vi "Multiplot-Disable.vi"() -> ()   [LabVIEW 2014]
uses:
  Stop.ctl
panel:
  in  "stop":T1
  in  "OK Button 3":bool
  in  "OK Button 2":bool
  in  "OK Button":bool
  out "Waveform Graph":dynamicdata(graph)
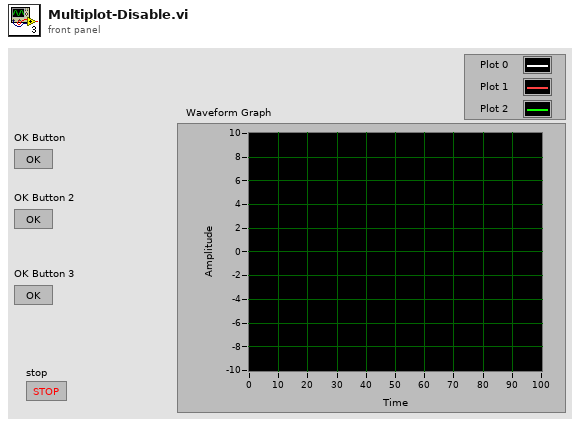
[diagram p1: front panel]
types:
  T1 = typedef "Stop.ctl" = bool
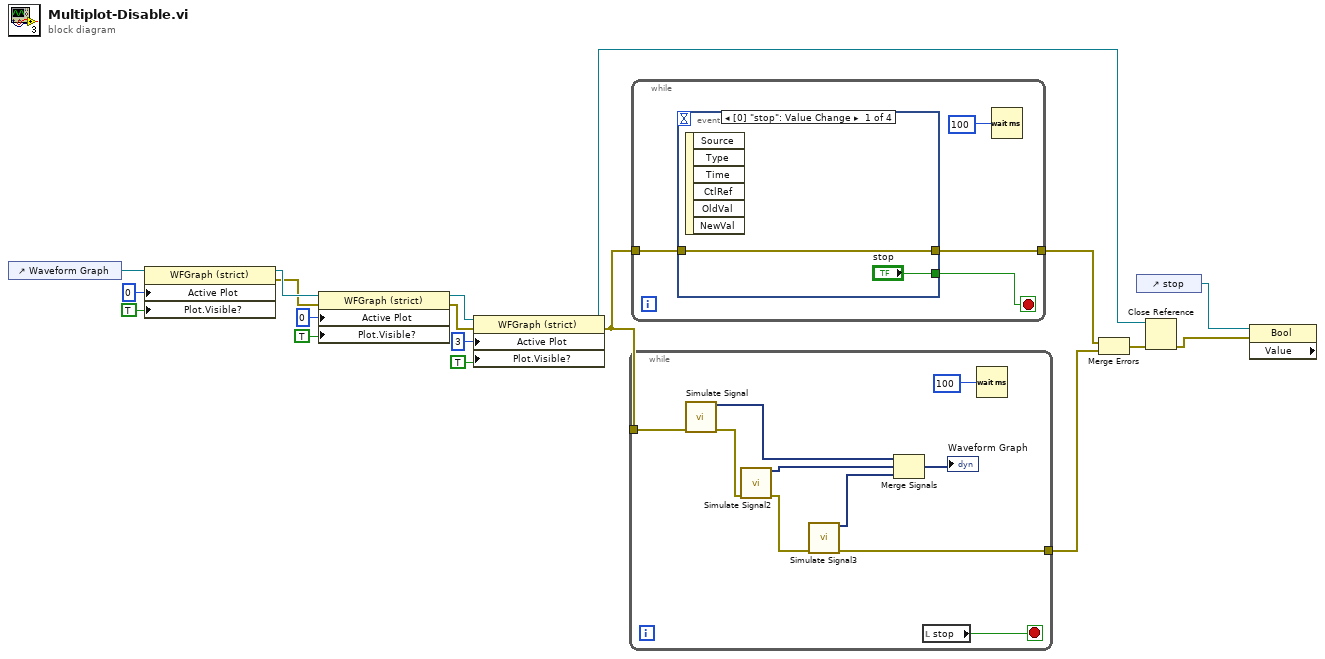
[diagram p0: block diagram]
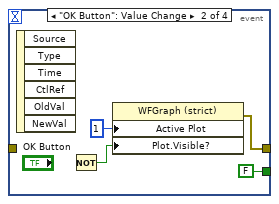
[diagram p2: hidden frame]
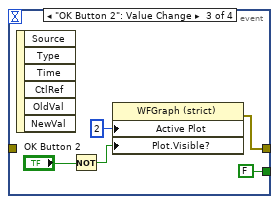
[diagram p3: hidden frame]
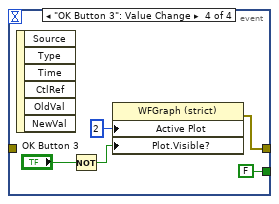
[diagram p4: hidden frame]
diagram:
  n1 = control-ref of="Waveform Graph"() -> (w18:refnum<vi>)
  n2 = property class="WFGraph (strict)"(reference=w18, "Active Plot"=u32 0, "Plot.Visible?"=TRUE ("Plot.Visible")) -> (reference out=w15:refnum<vi>, error out=w14:errorcluster)  [unwired: 1 in]
  n3 = property class="WFGraph (strict)"(reference=w15, error in=w14, "Active Plot"=u32 0, "Plot.Visible?"=TRUE ("Plot.Visible")) -> (reference out=w10:refnum<vi>, error out=w11:errorcluster)
  n4 = property class="WFGraph (strict)"(reference=w10, error in=w11, "Active Plot"=u32 3, "Plot.Visible?"=TRUE ("Plot.Visible")) -> (reference out=w3:refnum<vi>, error out=w6:errorcluster)
  n5 = while {
    tunnel: w6 -> [w27]
    tunnel: [w20] -> w5
    stop <- w19 stop-if-true
    n6 = call "Simulate Signal"("error in (no error)"=w27) -> ("Sine"=w24:dynamicdata, "error out"=w26:errorcluster)  [unwired: 13 in]
    n7 = call "Simulate Signal2"("error in (no error)"=w26) -> ("Square"=w23:dynamicdata, "error out"=w25:errorcluster)  [unwired: 13 in]
    n8 = call "Simulate Signal3"("error in (no error)"=w25) -> ("Triangle"=w22:dynamicdata, "error out"=w20:errorcluster)  [unwired: 13 in]
    n9 = Merge Signals(w24, w23, w22) -> (→"Waveform Graph":dynamicdata)
    n10 = local read "stop"() -> (w19:T1)
    n11 = Wait (ms)(milliseconds to wait=u32 100 ("millisecond timer value")) -> ()  [unwired: 1 out]
  }
  n12 = while {
    tunnel: w6 -> [w31]
    tunnel: [w29] -> w7
    stop <- w30 stop-if-true
    n13 = event shown="[0] \"stop\": Value Change" {
      selector: _ -> [_ _ _ _]
      dyn-events: _ -> [_ _ _ _]
      timeout: _ -> [_ _ _ _]
      tunnel: w31 -> [w33 _ _ _]
      tunnel: ["stop" FALSE ("stop") FALSE ("stop") FALSE ("stop")] -> w30
      tunnel: [w33 w35 w40 w45] -> w29
      event Value Change {
        n14 = event-data() -> ()  [unwired: 1 in, 6 out]
      }
      event "OK Button": Value Change {
        n15 = event-data() -> ()  [unwired: 1 in, 6 out]
        n16 = Not() -> (.not. x?=w37:bool)  [unwired: 1 in]
        n17 = property class="WFGraph (strict)"("Active Plot"=u32 1, "Plot.Visible?"=w37) -> (error out=w35:errorcluster)  [unwired: 2 in, 1 out]
      }
      event "OK Button 2": Value Change {
        n18 = event-data() -> ()  [unwired: 1 in, 6 out]
        n19 = Not(x="OK Button 2") -> (.not. x?=w42:bool)
        n20 = property class="WFGraph (strict)"("Active Plot"=u32 2, "Plot.Visible?"=w42) -> (error out=w40:errorcluster)  [unwired: 2 in, 1 out]
      }
      event "OK Button 3": Value Change {
        n21 = event-data() -> ()  [unwired: 1 in, 6 out]
        n22 = Not(x="OK Button 3") -> (.not. x?=w47:bool)
        n23 = property class="WFGraph (strict)"("Active Plot"=u32 2, "Plot.Visible?"=w47) -> (error out=w45:errorcluster)  [unwired: 2 in, 1 out]
      }
    }
    n24 = Wait (ms)(milliseconds to wait=u32 100 ("millisecond timer value")) -> ()  [unwired: 1 out]
  }
  n25 = Merge Errors(w7, w5) -> (w4:errorcluster)
  n26 = control-ref of="stop"() -> (w2:refnum<vi>)
  n27 = Close Reference(reference=w3, error in (no error)=w4) -> (error out=w1:errorcluster)
  n28 = property class="Bool" props=["Value"](reference=w2, error in=w1) -> ()  [unwired: 3 out]
